vi "Send onError.vi"(8 "error in (no error)":errorcluster, 10 "error to report":errorcluster, 11 "id":i32) -> (0 "error out":errorcluster)   [LabVIEW 2020, in "MCP Server.lvlib"]
uses:
  MCP Server.lvlib
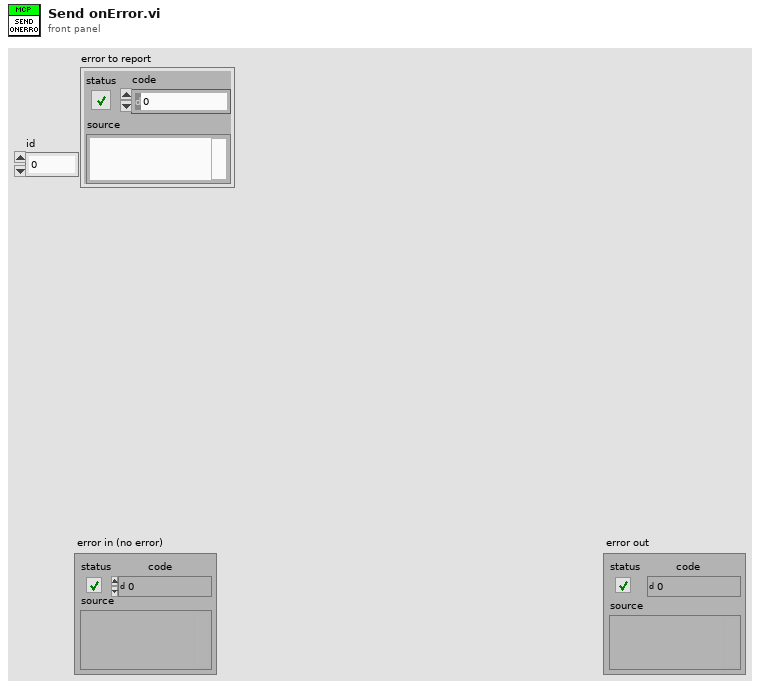
[diagram p1: front panel]
types:
  T1 = typedef "MCP Server.lvlib/Server Data.ctl" = cluster{"Name":string, "Description":string, "Tools":T2[], "Parameters":string[][], "Logging Info":T5, "User Events":T6, "Prompts":T7[], "resources":T9[], "HTTP Server":refnum<class "Server.lvclass">}
  T2 = typedef "MCP Server.lvlib/Tool Data.ctl" = cluster{"Name":string, "Description":string, "Ignored":string[], "inputs":T3[], "outputs":T4[], "VI Refnum":refnum<vi>}
  T3 = typedef "MCP Server.lvlib/Input Parameter.ctl" = cluster{"name":string, "type":string, "description":string, "required":bool, "raw name":string}
  T4 = typedef "MCP Server.lvlib/Output Parameter.ctl" = cluster{"name":string, "description":string, "type":string, "raw name":string}
  T5 = typedef "MCP Server.lvlib/Logging.ctl" = cluster{"Log":string[], "Max Length":i32}
  T6 = typedef "MCP Server.lvlib/User Events.ctl" = cluster{"onError":refnum<user-event>, "onRpc":refnum<user-event>}
  T7 = typedef "MCP Server.lvlib/Prompt Data.ctl" = cluster{"name":string, "description":string, "arguments":T8[], "return terminal name":string, "results description":string, "VI Refnum":refnum<vi>}
  T8 = typedef "MCP Server.lvlib/Prompt Argument.ctl" = cluster{"name":string, "description":string, "required":bool, "raw_name":string}
  T9 = typedef "MCP Server.lvlib/resource data.ctl" = cluster{"uri":string, "name":string, "description":string, "mimeType":string, "file path":path}
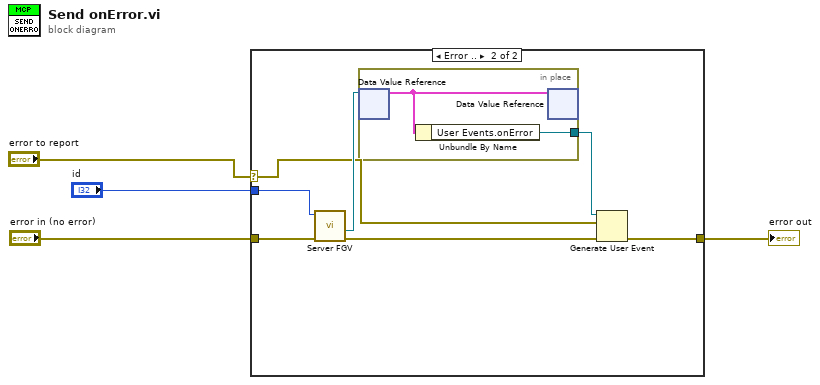
[diagram p0: block diagram]
diagram:
  n1 = case shown="Error .." "error to report" {
    selector: "error to report" -> [_ w6]
    tunnel: "error in (no error)" -> [w5 w12]
    tunnel: "id" -> [_ w10]
    tunnel: [w5 w9] -> w2
    frame No Error {
    }
    frame Error {
      n2 = call "Server FGV.vi"("error in"=w12, "id"=w10) -> ("error out"=w11:errorcluster, "server reference"=w8:refnum<data-value>)  [unwired: 5 in, 3 out]
      n3 = in-place {
        in-place-border: [w13] -> w7
        n4 = in-place-dvr #1(w8) -> (w14:T1)  [unwired: 1 out]
        n5 = Unbundle By Name(w14) -> ("User Events.onError"=w13:refnum<user-event>)
        n6 = in-place-dvr #1(w14) -> ()  [unwired: 2 out]
      }
      n7 = Generate User Event(user event=w7, event data cluster=w6, error in=w11) -> (error out=w9:errorcluster)  [unwired: 1 in, 1 out]
    }
  }
  "error out" <- w2
